vi "Cross_Correlation.vi"() -> (5 "Plug in titles":string[](array[string]), 7 "Plug in values":string[](array[string]))   [LabVIEW 2012]
uses:
  Globals/Meas_global.vi
panel:
  out "XY Graph":cluster{dbl[], dbl[]}[](graph)
  in  "Time window half width":dbl=3.0
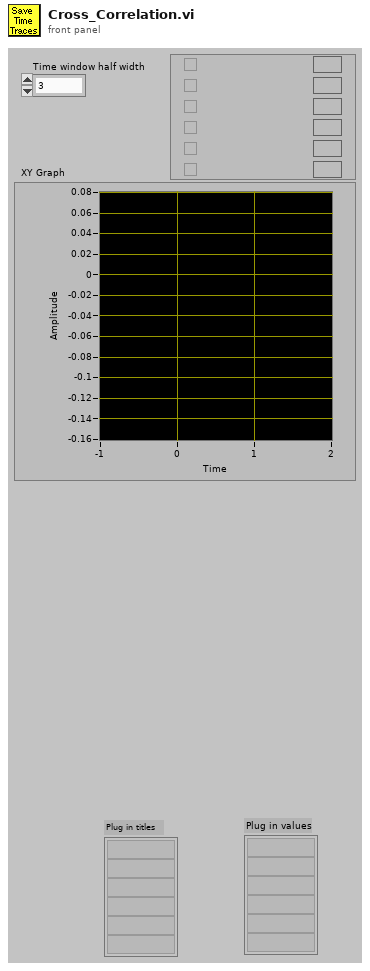
[diagram p1: front panel]
types:
  T1 = typedef "Time_Trace_Cluster.ctl" = cluster{"Weighting":dbl[], "Time (s)":dbl[], "Voltage":dbl[], "Eng Values":dbl[]}
  T2 = typedef "Analysis_info_cluster.ctl" = cluster{"Colour":u32, "Inst type":T3, "Inst name":string, "Symbol":string, "Code name":string, "Extra Info":string, "Inst Array":T4, "Extra Titles":string[], "Extra Values":string[], "U":dbl, "u^2":dbl, "u^3":dbl, "u^4":dbl, "Skew_u":dbl, "Kurt_u":dbl, "Sd Error in Mean":dbl, "% u'/U":dbl, "X":dbl, "Y":dbl, "Z":dbl, "Timescale integral to 25%":dbl, "Sd Error in Variance":dbl, "Calib File":path, "Calib Constants":dbl[], "Output Position":bool, "Full Stats":bool, "Av Sampling Rate":dbl, "Av No of Samples":dbl, "Total Meas Time (s)":dbl, "ADAM Ch Name":string}
  T3 = typedef "Inst_type.ctl" = enum16{"Propeller anemometer", "Raw voltage", "Pressure Transducer", "Pitot-static tube", "Preston tube", "Hot wire", "Cross wire 1", "Cross wire 2", "Generic Linear", "Generic Polynomial", "Generic BackPoly", "Fast FID", "Thermocouple", "Cold wire", "Pulsed Wire", "LDA Vel", "LDA Tran time", "LDA Arr time"}
  T4 = typedef "Instrument_Array.ctl" = enum16{"PWA", "LDA", "Analogue"}
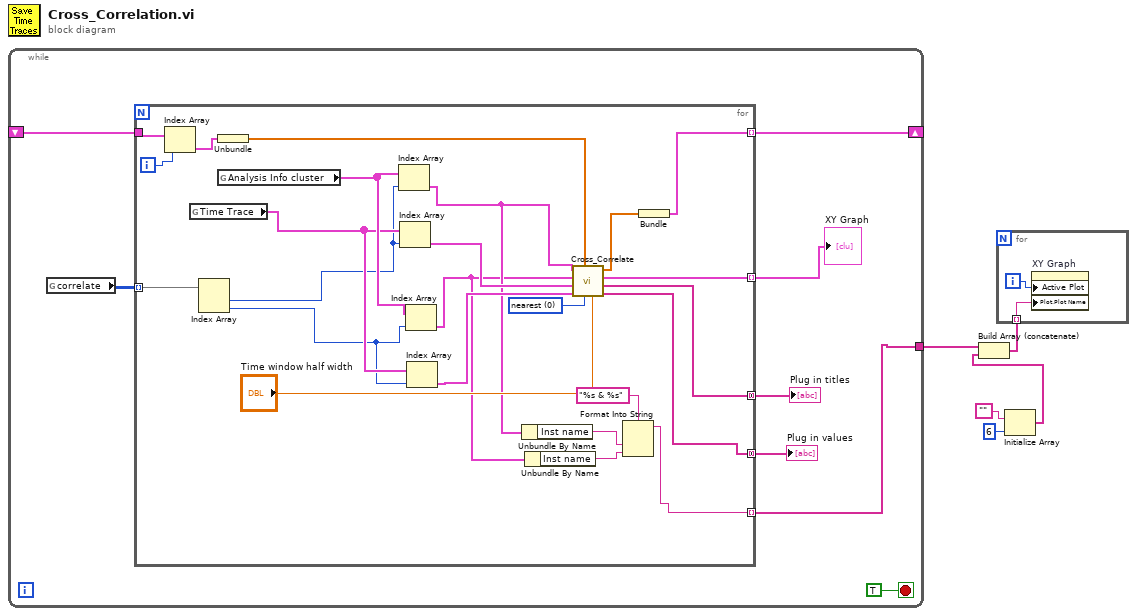
[diagram p0: block diagram]
diagram:
  n1 = while {
    shift-right: [w12] -> _
    shift-left: _ -> [w11]
    tunnel: [w6] -> w3
    stop <- TRUE stop-if-true
    n2 = global read "Meas_global.vi" "correlate"() -> (w13:i32[][])
    n3 = for {
      tunnel: w13 -> [w32] mode=indexing
      tunnel: [w27] -> w12 mode=indexing
      tunnel: w11 -> [w25]
      tunnel: [w21] -> w9 mode=concatenating
      tunnel: [w23] -> w10 mode=indexing
      tunnel: [w22] -> w8 mode=concatenating
      tunnel: [w14] -> w6 mode=indexing
      i -> [w15]
      w33 = 0 items=["nearest", "linear", "spline", "cubic Hermite", "Lagrange"] ("interp. method")
      n4 = Index Array(array=w25, index=w15) -> (element=w24:cluster{"Shift output array":dbl[]})
      n5 = global read "Meas_global.vi" "Time Trace"() -> (w36:T1[])
      n6 = Index Array(array=w32) -> (element #1=w31:i32, element #2=w30:i32)  [unwired: 2 in]
      n7 = Unbundle(w24) -> ("Shift output array"=w26:dbl[])
      n8 = global read "Meas_global.vi" "Analysis Info cluster"() -> (w37:T2[])
      n9 = Index Array(array=w37, index=w31) -> (element=w20:T2)
      n10 = Index Array(array=w36, index=w31) -> (element=w35:T1)
      n11 = Index Array(array=w37, index=w30) -> (element=w19:T2)
      n12 = Index Array(array=w36, index=w30) -> (element=w34:T1)
      n13 = Unbundle By Name(w20) -> ("Inst name"=w18:string)
      n14 = Unbundle By Name(w19) -> ("Inst name"=w17:string)
      n15 = call "Cross_Correlate.vi"("Time window half width"="Time window half width", "interp. method"=w33, "Shift input array"=w26, "Time Cluster 2"=w34, "Time Cluster 1"=w35, "Cluster 2"=w19, "Cluster 1"=w20) -> ("Plug In Values"=w21:string[], "Plug In Titles"=w22:string[], "XY Graph"=w23:cluster{dbl[], dbl[]}, "Shift output array"=w28:dbl[])  [unwired: 1 in]
      n16 = Format Into String(format string="%s & %s", w18, w17) -> (resulting string=w14:string)  [unwired: 2 in, 1 out]
      n17 = Bundle("Shift output array"=w28) -> (w27:cluster{"Shift output array":dbl[]})  [unwired: 1 in]
    }
    "Plug in titles" <- w8
    "Plug in values" <- w9
    "XY Graph" <- w10
  }
  n18 = Initialize Array("", 6 ("dimension size")) -> (w2:string[])
  n19 = Build Array (concatenate)(w3, w2) -> (w1:string[])
  n20 = for {
    tunnel: w1 -> [w39] mode=indexing
    i -> [w38]
    n21 = property on="XY Graph" class="XYGraph (strict)"("Active Plot"=w38, "Plot.Plot Name"=w39) -> ()  [unwired: 2 in, 2 out]
  }
